vi "PH_OceanOpticsSpectrometer.evt call Remote Control.vi"(0 "i ref in":refnum<vi>, 2 "Instance":string="N/A", 3 "Control Remote?":bool, 5 "error in (no error)":errorcluster) -> (14 "i ref out":refnum<vi>, 19 "error out":errorcluster)   [LabVIEW 2014, in "PH_OceanOpticsSpectrometer.lvlib"]
doc: "This VI sends a comand by a simple call."
uses:
  PH_OceanOpticsSpectrometer.lvlib
  CSCore/CSSystem/CoreLib/CoreLib.short 2 byte array.vi
  CSCore/CSSystem/CoreLib/CoreLib.lvlib
  CSCore/BaseProcess/BaseProcess.lvlib
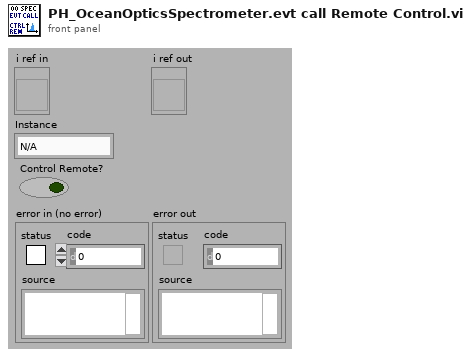
[diagram p1: front panel]
types:
  T1 = typedef "CoreDefs.rawDataType.ctl" = i8[]
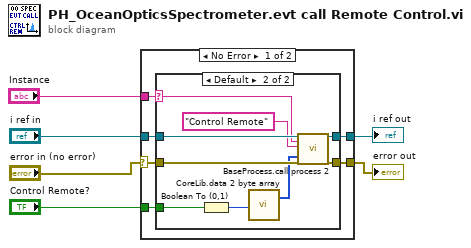
[diagram p0: block diagram]
diagram:
  n1 = case shown="No Error" "error in (no error)" {
    selector: "error in (no error)" -> [w8 w24]
    tunnel: [w12 w25] -> w2
    tunnel: [w11 w24] -> w3
    tunnel: "i ref in" -> [w10 w25]
    tunnel: "Instance" -> [w9 _]
    tunnel: "Control Remote?" -> [w7 _]
    frame No Error {
      n2 = case shown="Default" w9 {
        selector: w9 -> [_ w16]
        tunnel: [w14 w23] -> w12
        tunnel: [w13 w22] -> w11
        tunnel: w10 -> [w14 w21]
        tunnel: w8 -> [w13 w20]
        tunnel: w7 -> [_ w15]
        frame "N/A" {
        }
        frame Default {
          n3 = Boolean To (0,1)(Boolean=w15) -> (0, 1=w18:i16)
          n4 = call-poly "CoreLib.data 2 byte array.vi"("i16"=w18) -> ("byteArray out"=w17:T1)  [unwired: 18 in]
          n5 = call "BaseProcess.call process 2.vi"("i ref in"=w21, "Object"=w16, "Selector"="Control Remote", "Data"=w17, "error in (no error)"=w20) -> ("i ref out"=w23:refnum<vi>, "error out"=w22:errorcluster)  [unwired: 13 in]
        }
      }
    }
    frame Error {
    }
  }
  "error out" <- w3
  "i ref out" <- w2
